vi "Thermal_Camera_Stream.vi"() -> ()   [LabVIEW 2020]
uses:
  <vilib>/userDefined/High Color/IMAQdx.ctl
  <vilib>/vision/driver/NI_Vision_Acquisition_Software.lvlib
  <resource>/objmgr/imaqdx.rc
  <vilib>/vision/NI_Vision_Development_Module.lvlib
panel:
  out "Intensity Graph 2":i8[][](graph)
  in  "sample size":i32=2
  out "period (ms)":u32
  in  "a65?":bool=TRUE
  out "error out":errorcluster
  out "Temperature":dbl
  out "Image":T1(plugin-control)
  in  "Stop":bool
  in  "Session In":T2="cam4"
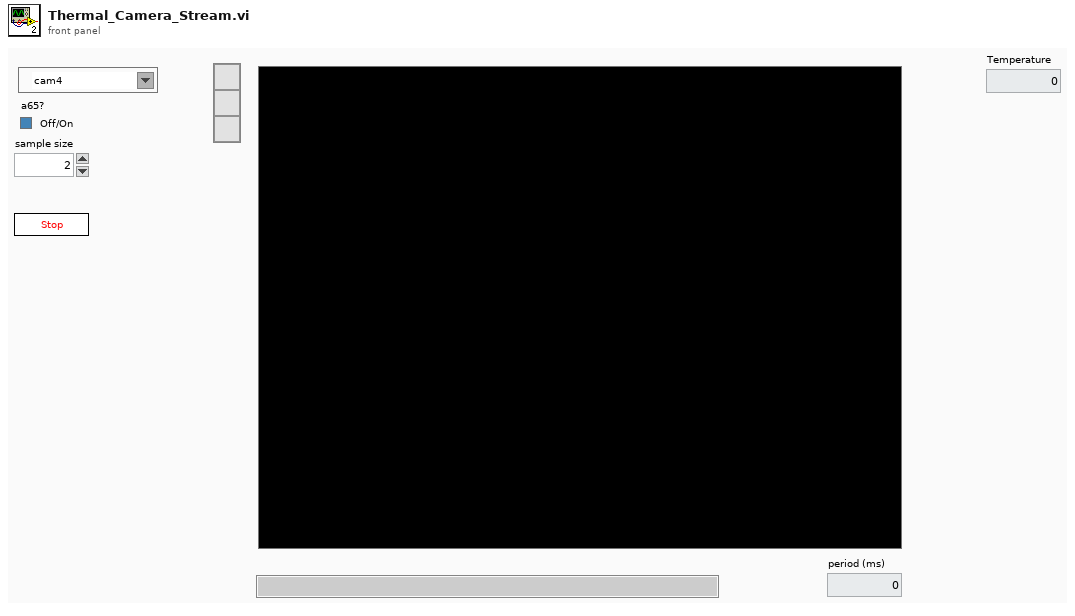
[diagram p1: front panel]
types:
  T1 = typedef "IMAQ Image.ctl" = refnum<image>
  T2 = typedef "IMAQdx.ctl" = refnum<k21>
  T3 = typedef "Image Type" = u32
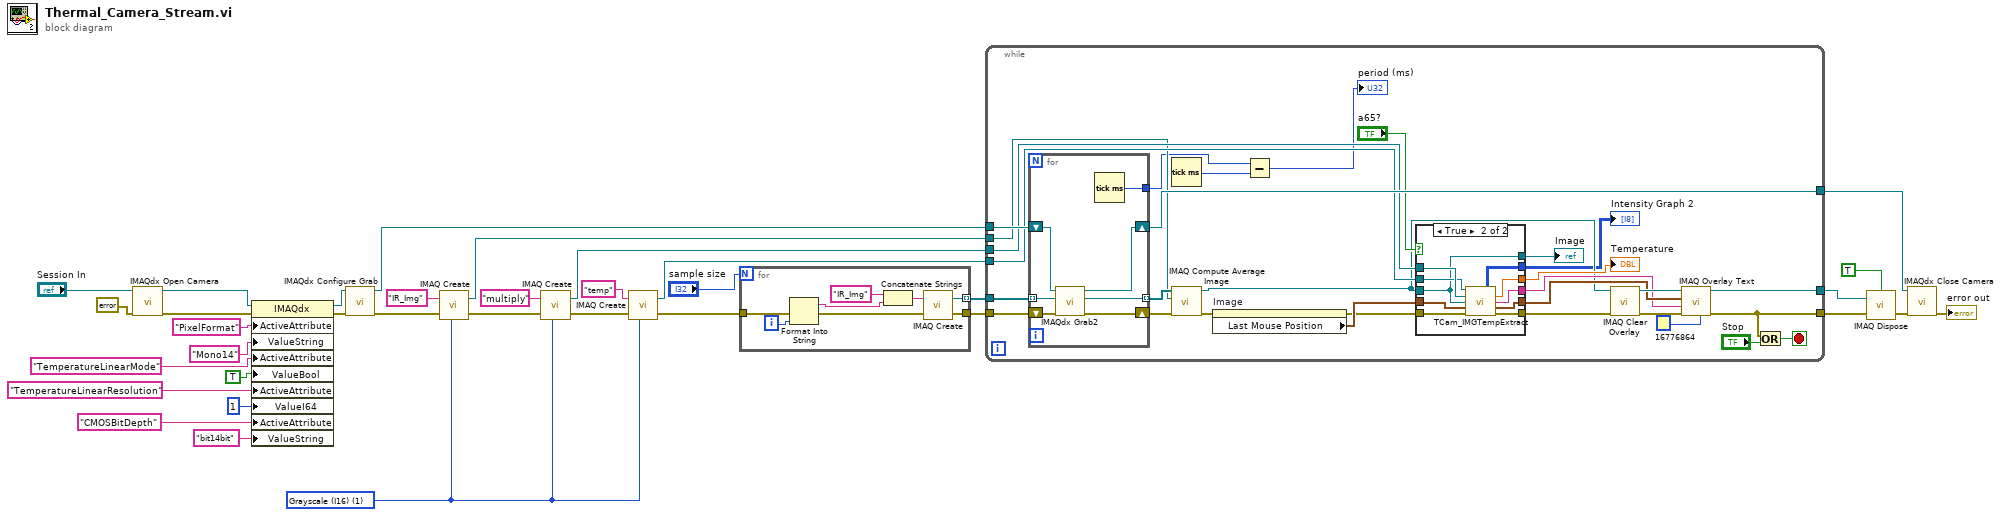
[diagram p0: block diagram]
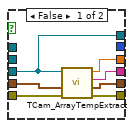
[diagram p2: hidden frame]
diagram:
  w11 = T3 1 items=["Grayscale (U8)", "Grayscale (I16)", "Grayscale (SGL)", "Complex (CSG)", "RGB (U32)", "HSL (U32)", "RGB (U64)", "Grayscale (U16)"] ("Image Type")
  n1 = call <vilib>:"IMAQdx Open Camera.vi"("error in"=errorcluster {"status"=FALSE, "code"=0, "source"=""}, "Session In"="Session In") -> ("error out"=w34:errorcluster, "Session Out"=w35:T2)  [unwired: 8 in]
  n2 = property class="IMAQdx"(reference=w35, error in=w34, "ActiveAttribute"="PixelFormat", "ValueString"="Mono14", "ActiveAttribute"="TemperatureLinearMode", "ValueBool"=TRUE, "ActiveAttribute"="TemperatureLinearResolution", "ValueI64"=i64 1, "ActiveAttribute"="CMOSBitDepth", "ValueString"="bit14bit") -> (reference out=w28:T2, error out=w27:errorcluster)
  n3 = call <vilib>:"IMAQdx Configure Grab.vi"("error in"=w27, "Session In"=w28) -> ("error out"=w25:errorcluster, "Session Out"=w26:T2)  [unwired: 8 in]
  n4 = call "IMAQ Create"("Image Name"="IR_Img", "Image Type"=w11, "error in (no error)"=w25) -> ("New Image"=w24:T1, "error out"=w8:errorcluster)  [unwired: 2 in]
  n5 = call "IMAQ Create"("Image Name"="multiply", "Image Type"=w11, "error in (no error)"=w8) -> ("New Image"=w6:T1, "error out"=w7:errorcluster)  [unwired: 2 in]
  n6 = call "IMAQ Create"("Image Name"="temp", "Image Type"=w11, "error in (no error)"=w7) -> ("New Image"=w5:T1, "error out"=w2:errorcluster)  [unwired: 2 in]
  n7 = for {
    N: "sample size" -> [_]
    tunnel: [w39] -> w4 mode=indexing
    tunnel: w2 -> [w38]
    tunnel: [w36] -> w1
    i -> [w41]
    n8 = Format Into String(error in=w38, w41) -> (resulting string=w40:string, error out=w37:errorcluster)  [unwired: 2 in]
    n9 = Concatenate Strings("IR_Img" ("Image Name"), w40) -> (w42:string)
    n10 = call "IMAQ Create"("Image Name"=w42, "error in (no error)"=w37) -> ("New Image"=w39:T1, "error out"=w36:errorcluster)  [unwired: 3 in]
  }
  n11 = while {
    tunnel: w26 -> [w71]
    tunnel: w1 -> [w70]
    tunnel: w24 -> [w51]
    tunnel: [w67] -> w23
    tunnel: [w65] -> w22
    tunnel: [w64] -> w20
    tunnel: w6 -> [w63]
    tunnel: w5 -> [w62]
    tunnel: w4 -> [w54]
    stop <- w72 stop-if-true
    n12 = for {
      shift-right: [w78] -> w64
      shift-left: w71 -> [w80]
      shift-right: [w77] -> w52
      shift-left: w70 -> [w79]
      tunnel: w54 -> [w76] mode=indexing
      tunnel: [w75] -> w53 mode=indexing
      tunnel: [w74] -> w47
      n13 = call <vilib>:"IMAQdx Grab2.vi"("error in"=w79, "Image In"=w76, "Session In"=w80) -> ("error out"=w77:errorcluster, "Image Out"=w75:T1, "Session Out"=w78:T2)  [unwired: 5 in, 1 out]
      n14 = Tick Count (ms)() -> (millisecond timer value=w74:u32)
    }
    n15 = Tick Count (ms)() -> (millisecond timer value=w48:u32)
    n16 = call "IMAQ Compute Average Image"("error in (no error)"=w52, "Image Dst"=w51, "Images"=w53) -> ("error out"=w49:errorcluster, "Image Dst Out"=w50:T1)  [unwired: 7 in]
    n17 = property on="Image" class="ImageControl"(error in=w49) -> (error out=w58:errorcluster, "Last Mouse Position"=w59:cluster{"X":i32, "Y":i32})  [unwired: 1 in, 1 out]
    n18 = Subtract(x=w47, y=w48) -> (x-y=→"period (ms)":u32)
    n19 = case shown="True" "a65?" {
      tunnel: w50 -> [w87 w89]
      tunnel: w63 -> [_ w97]
      tunnel: w62 -> [_ w96]
      tunnel: w58 -> [w86 w95]
      tunnel: [w85 w94] -> w61
      tunnel: [w84 w93] -> w60
      tunnel: [w87 w89] -> w45
      tunnel: w59 -> [w83 w92]
      tunnel: [w82 w91] -> w57
      tunnel: [w81 w90] -> w55
      tunnel: [_ w88] -> w44
      frame False {
        n20 = call "TCam_ArrayTempExtract.vi"("error in (no error)"=w86, "Mouse pos"=w83, "img in"=w87) -> ("error out"=w84:errorcluster, "Mouse pos dup"=w82:cluster{"X":i32, "Y":i32}, "temp str"=w81:string, "temp"=w85:dbl)  [unwired: 5 in]
      }
      frame True {
        n21 = call "TCam_IMGTempExtract.vi"("img dst"=w96, "img process dst"=w97, "Image in"=w89, "Mouse pos"=w92, "error in (no error)"=w95) -> ("appended array"=w88:i8[][], "temp"=w94:sgl, "temp str"=w90:string, "Mouse pos dup"=w91:cluster{"X":i32, "Y":i32}, "error out"=w93:errorcluster)  [unwired: 5 in, 1 out]
      }
    }
    "Temperature" <- w61
    "Image" <- w45
    "Intensity Graph 2" <- w44
    n22 = call "IMAQ Clear Overlay"("error in (no error)"=w60, "Image"=w50) -> ("error out"=w66:errorcluster, "Image Out"=w68:T1)  [unwired: 8 in]
    n23 = call "IMAQ Overlay Text"("BG Color (Transparent)"=u32 16776864, "error in (no error)"=w66, "String"=w55, "Origin"=w57, "Image"=w68) -> ("error out"=w65:errorcluster, "Image Out"=w67:T1)  [unwired: 5 in]
    n24 = Or(x=w65, y="Stop") -> (x .or. y?=w72:bool)
  }
  n25 = call "IMAQ Dispose"("All Images? (No)"=TRUE, "Image"=w23, "error in (no error)"=w22) -> ("error out"=w21:errorcluster)  [unwired: 3 in]
  n26 = call <vilib>:"IMAQdx Close Camera.vi"("error in"=w21, "Session In"=w20) -> ("error out"=→"error out":errorcluster)  [unwired: 9 in]
